vi "SECoP_dataGetArrayLength.vi"(7 "Position":u32, 8 "error in (no error)":errorcluster, 10 "SECoP_dataPtr":T1 {"ptr64" format="%.0x"; "ptr32" format="%.0x"}, 11 "DLL path (in)":T2) -> (0 "error out":errorcluster, 2 "array length":u32, 3 "DLL path (out)":T2, 4 "maximum length":u32, 5 "minimum length":u32)   [LabVIEW 2023, in "SECoP.lvlib"]
doc: "Call <b>\"SECoP_dataGetArrayLength.vi\"</b> to return the length of an array (SECoP_dataPtr).\n\n<b>DLL path</b> input and output of cluster from \"SECoP-Initialize.vi\"\n<b>SECoP_dataPtr</b> data to access\n<b>Position</b> points to a virtual flattened entry of the data type\n<b>array length</b> actual length of the array\n<b>minimum length</b> minimum allowed length\n<b>maximum length</b> maximum allowed length"
uses:
  SECoP.lvlib
  SECoP-libraries.ctl
  SECoP-data.ctl
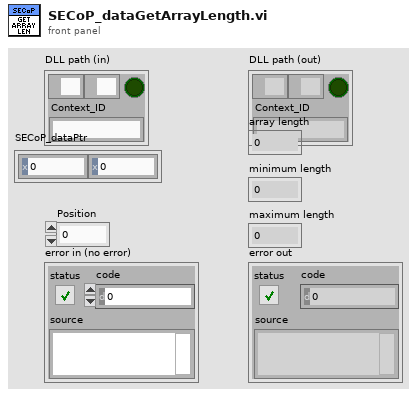
[diagram p1: front panel]
types:
  T1 = typedef "SECoP.lvlib/SECoP-data.ctl" = cluster{"ptr32":u32, "ptr64":u64}
  T2 = typedef "SECoP.lvlib/SECoP-libraries.ctl" = cluster{"serverDLL":path, "variantDLL":path, "cleanup_mode":bool, "Context_ID":string}
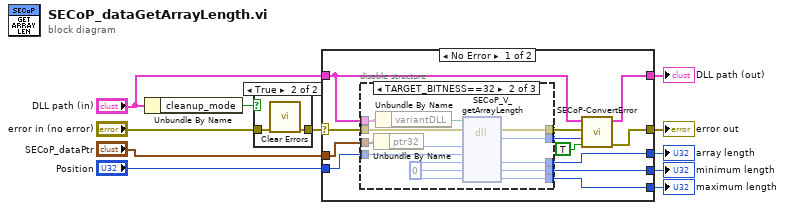
[diagram p0: block diagram]
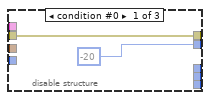
[diagram p3: hidden frame]
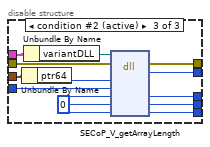
[diagram p4: hidden frame]
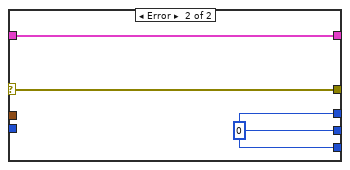
[diagram p5: hidden frame]
diagram:
  n1 = Unbundle By Name("DLL path (in)") -> ("cleanup_mode"=w9:bool)
  n2 = case shown="True" w9 {
    tunnel: "error in (no error)" -> [w12 w14]
    tunnel: [w12 w13] -> w7
    frame False {
    }
    frame True {
      n3 = call <vilib>:"Clear Errors.vi"("error in (no error)"=w14) -> ("error out"=w13:errorcluster)  [unwired: 5 in, 1 out]
    }
  }
  n4 = case shown="No Error" w7 {
    selector: w7 -> [w24 w54]
    tunnel: "DLL path (in)" -> [w15 w55]
    tunnel: [w25 w55] -> w11
    tunnel: [w26 w54] -> w10
    tunnel: "Position" -> [w20 _]
    tunnel: [w19 w53] -> w5
    tunnel: "SECoP_dataPtr" -> [w18 _]
    tunnel: [w17 w53] -> w3
    tunnel: [w16 w53] -> w2
    frame No Error {
      n5 = disable-structure shown="TARGET_BITNESS==32" {
        disable-tunnel: w24 -> [w28 w40 w52]
        disable-tunnel: w15 -> [_ w39 w51]
        disable-tunnel: [w28 w38 w50] -> w23
        disable-tunnel: [-20 w37 w49] -> w22
        disable-tunnel: w20 -> [_ w36 w48]
        disable-tunnel: [_ w32 w44] -> w19
        disable-tunnel: w18 -> [_ w34 w46]
        disable-tunnel: [_ w31 w43] -> w17
        disable-tunnel: [_ w30 w42] -> w16
        frame condition #0 {
        }
        frame condition #1 {
          w33 = u32 0 ("uLength")
          n6 = Unbundle By Name(w34) -> ("ptr32"=w35:u32)
          n7 = Unbundle By Name(w39) -> ("variantDLL"=w29:path)
          n8 = dll-call lib="Z:/Praktische_Aufgaben/SECoP-LabVIEW2015/32bit/SECoP32.dll" fn="SECoP_V_getArrayLength"(path in=w29, error in=w40, "pData"=w35, "uPosition"=w36, "uLength"=w33, "uMinimumLength"=w33, "uMaximumLength"=w33) -> (error out=w38:errorcluster, "return type"=w37:i32, "uLength"=w30:u32, "uMinimumLength"=w31:u32, "uMaximumLength"=w32:u32)  [unwired: 3 in, 1 out]
        }
        frame condition #2 (active) {
          w45 = u32 0 ("uLength")
          n9 = Unbundle By Name(w46) -> ("ptr64"=w47:u64)
          n10 = Unbundle By Name(w51) -> ("variantDLL"=w41:path)
          n11 = dll-call lib="Z:/Praktische_Aufgaben/SECoP-LabVIEW2015/32bit/SECoP32.dll" fn="SECoP_V_getArrayLength"(path in=w41, error in=w52, "pData"=w47, "uPosition"=w48, "uLength"=w45, "uMinimumLength"=w45, "uMaximumLength"=w45) -> (error out=w50:errorcluster, "return type"=w49:i32, "uLength"=w42:u32, "uMinimumLength"=w43:u32, "uMaximumLength"=w44:u32)  [unwired: 3 in, 1 out]
        }
      }
      n12 = call "SECoP-ConvertError.vi"("return is boolean"=TRUE, "return code"=w22, "error in (no error)"=w23, "DLL path (in)"=w15) -> ("error out"=w26:errorcluster, "DLL path (out)"=w25:T2)  [unwired: 6 in]
    }
    frame Error {
      w53 = u32 0 ("Value")
    }
  }
  "DLL path (out)" <- w11
  "error out" <- w10
  "maximum length" <- w5
  "minimum length" <- w3
  "array length" <- w2
